vi "Register to Discovery Service.vi"(8 "error in":errorcluster, 9 "Measurement":refnum<class "MeasurementPluginService.lvclass">, 10 "PortNumber":i32, 11 "gRPC ID":T2) -> (0 "error out":errorcluster, 2 "Response Data":T1, 3 "gRPC ID out":T2)   [LabVIEW 2020, in "MeasurementLink Measurement Server.lvlib"]
uses:
  MeasurementLink Measurement Server.lvlib
  <vilib>/gRPC/LabVIEW gRPC Library/Shared/grpcId.ctl
  <vilib>/MeasurementLink/Discovery Client/RPC Messages/ni_measurementlink_discovery_v1_RegisterServiceResponse.ctl
  Classes/MeasurementPluginService/MeasurementPluginService.lvclass
  <vilib>/MeasurementLink/Discovery Client/RPC Messages/ni_measurementlink_discovery_v1_RegisterServiceRequest.ctl
  <vilib>/MeasurementLink/Discovery Client/RPC Messages/ni_measurementlink_discovery_v1_ServiceDescriptor.ctl
  <vilib>/MeasurementLink/Discovery Client/RPC Messages/ni_measurementlink_discovery_v1_ServiceLocation.ctl
  <vilib>/MeasurementLink/Discovery Client/MeasurementLink Discovery Client.lvlib
  <vilib>/gRPC/LabVIEW gRPC Library/grpc-lvsupport-release.lvlib
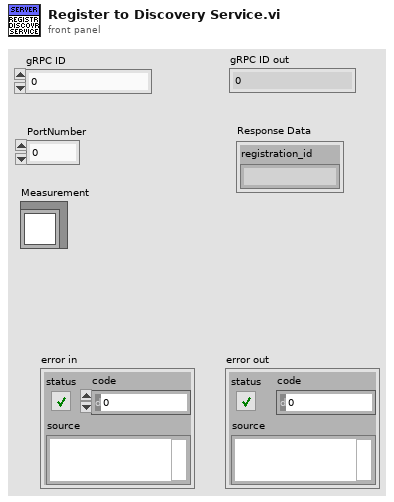
[diagram p1: front panel]
types:
  T1 = typedef "MeasurementLink Discovery Client.lvlib/ni_measurementlink_discovery_v1_RegisterServiceResponse.ctl" = cluster{"registration_id":string}
  T2 = typedef "grpc-lvsupport-release.lvlib/grpcId.ctl" = u64
  T3 = typedef "MeasurementLink Discovery Client.lvlib/ni_measurementlink_discovery_v1_RegisterServiceRequest.ctl" = cluster{"service_description":T4, "location":T5}
  T4 = typedef "MeasurementLink Discovery Client.lvlib/ni_measurementlink_discovery_v1_ServiceDescriptor.ctl" = cluster{"display_name":string, "description_url":string, "provided_interfaces":string[], "service_class":string}
  T5 = typedef "MeasurementLink Discovery Client.lvlib/ni_measurementlink_discovery_v1_ServiceLocation.ctl" = cluster{"location":string, "insecure_port":string, "ssl_authenticated_port":string}
  T6 = typedef "MeasurementLink Measurement Server Internal.lvlib/ni_measurementlink_measurement_v1_MeasurementDetails.ctl" = cluster{"display_name":string, "version":string}
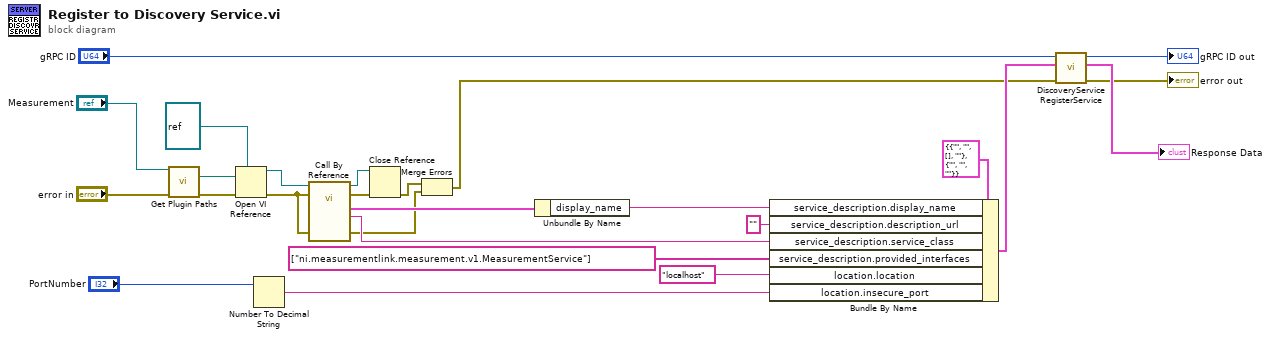
[diagram p0: block diagram]
diagram:
  n1 = call-dynamic "Get Plugin Paths.vi"("MeasurementService in"="Measurement", "error in (no error)"="error in") -> ("Get Measurement Details VI Path"=w2:path, "error out"=w3:errorcluster)  [unwired: 7 in, 5 out]
  n2 = Open VI Reference(type specifier VI Refnum (for type only)=refnum<vi> refnum, vi path=w2, error in (no error)=w3) -> (vi reference=w14:refnum<vi>, error out=w10:errorcluster)  [unwired: 3 in]
  n3 = Number To Decimal String(number="PortNumber") -> (decimal integer string=w26:string)  [unwired: 1 in]
  n4 = call-by-ref "?"(reference=w14, error in=w10, "error in"=w10) -> (reference out=w9:refnum<vi>, error out=w8:errorcluster, 0:"error out"=w6:errorcluster, "Service Class"=w11:string, "Measurement Details"=w12:T6)  [unwired: 8 in]
  n5 = Close Reference(reference=w9, error in (no error)=w8) -> (error out=w7:errorcluster)
  n6 = Merge Errors(w7, w6) -> (w5:errorcluster)
  n7 = Unbundle By Name(w12) -> ("display_name"=w22:string)
  n8 = Bundle By Name(cluster=T3 {"service_description"={"display_name"="", "description_url"="", "provided_interfaces"=[], "service_class"=""}, "location"={"location"="", "insecure_port"="", "ssl_authenticated_port"=""}} ("Request Data"), "service_description.display_name"=w22, "service_description.description_url"="", "service_description.service_class"=w11, "service_description.provided_interfaces"=string[] ["ni.measurementlink.measurement.v1.MeasurementService"] ("provided_services"), "location.location"="localhost", "location.insecure_port"=w26) -> (w19:T3)
  n9 = call <vilib>:"DiscoveryService RegisterService.vi"("error in"=w5, "Request Data"=w19, "gRPC ID"="gRPC ID") -> ("error out"=→"error out":errorcluster, "Response Data"=→"Response Data":T1, "gRPC ID out"=→"gRPC ID out":T2)  [unwired: 6 in]
